vi "Step4_2_LowPass.vi"(9 "s_axis_data_tdata":fxp<+/-,18,1>, 10 "s_axis_data_tvalid":bool) -> (1 "m_axis_data_tdata":fxp<+/-,40,1>, 2 "m_axis_data_tvalid":bool, 3 "s_axis_data_tready":bool)   [LabVIEW 2018]
uses:
  <vilib>/rvi/XilinxIP/XIPIN_XNode/niFpgaXIPIN.xnode
  Deprecated_Delete/DigitalFilterDesign/FIR_Filter_Configuration/FIR Compiler/xsim.dir/FIR_Compiler_3CE652926F5B43F18022D1349C670FA0/xsimk_3CE652926F5B43F18022D1349C670FA0.dll
  <vilib>/rvi/IPIntegrationNode/IPINode_Xnode/niFpgaIPINode.xnode
  <vilib>/rvi/IPIntegrationNode/IPINode_Typedef/niFpgaIPINodeSupportedFamilies.ctl
  <vilib>/rvi/IPIntegrationNode/IPINode_Utilities/niFpgaIPINodeSimCore.vi
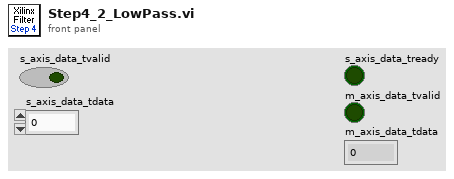
[diagram p1: front panel]
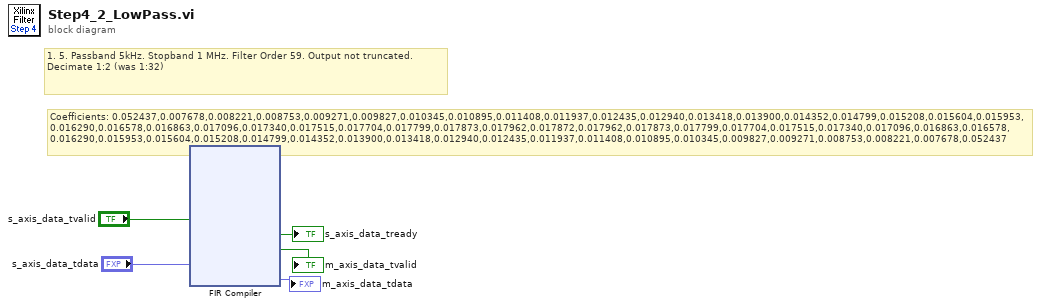
[diagram p0: block diagram]
diagram:
  # "Coefficients: 0.052437,0.007678,0.008221,0.008753,0.009271,0.009827,0.010345,0.010895,0.011408,0.011937,0.012435,0.012940,0.013418,0.013900,0.014352,0.014799,0.015208,0.015604,0.015953,\n0.016290,0.016578,0.016863,0.017096,0.017340,0.017515,0.017704,0.017799,0.017873,0.017962,0.017872,0.017962,0.017873,0.017799,0.017704,0.017515,0.017340,0.017096,0.016863,0.016578,\n0.016290,0.015953,0.015604,0.015208,0.014799,0.014352,0.013900,0.013418,0.012940,0.012435,0.011937,0.011408,0.010895,0.010345,0.009827,0.009271,0.008753,0.008221,0.007678,0.052437"
  # "1.\t5.\tPassband 5kHz. Stopband 1 MHz. Filter Order 59. Output not truncated.\nDecimate 1:2 (was 1:32)"
  n1 = xnode ("FIR Compiler")("s_axis_data_tvalid"="s_axis_data_tvalid", "s_axis_data_tdata"="s_axis_data_tdata") -> ("s_axis_data_tready"=→"s_axis_data_tready":bool, "m_axis_data_tvalid"=→"m_axis_data_tvalid":bool, "m_axis_data_tdata"=→"m_axis_data_tdata":fxp<+/-,40,1>)
